vi "Encoder State.vi"(8 "error in (no error)":errorcluster) -> (0 "error out":errorcluster, 2 "Gamma":dbl, 3 "Combined Wheel Angle":dbl)   [LabVIEW 2014]
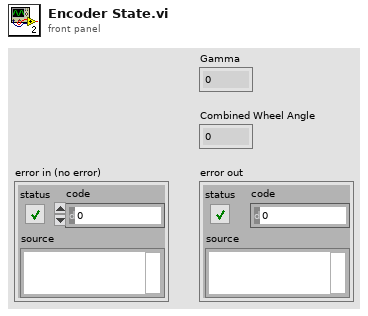
[diagram p1: front panel]
types:
  T1 = cluster{"Encoder 1":i32, "Encoder 2":i32, "Encoder 3":i32, "Encoder 4":i32}
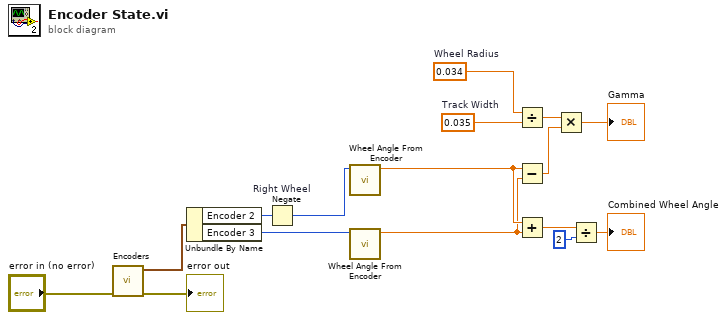
[diagram p0: block diagram]
diagram:
  w15 = 0.035  # Track Width
  w14 = 0.034  # Wheel Radius
  n1 = call "Encoders.vi"("error in (no error)"="error in (no error)") -> ("error out"=→"error out":errorcluster, "Encoder Data"=w3:T1)  [unwired: 9 in]
  n2 = Unbundle By Name(w3) -> ("Encoder 2"=w2:i32, "Encoder 3"=w1:i32)
  n3 = Negate "Right Wheel"(x=w2) -> (-x=w10:i32)
  n4 = call "Wheel Angle From Encoder.vi"("Numeric in"=w10) -> ("Numeric out"=w12:dbl)  [unwired: 10 in]
  n5 = call "Wheel Angle From Encoder.vi"("Numeric in"=w1) -> ("Numeric out"=w11:dbl)  [unwired: 10 in]
  n6 = Divide(x=w14, y=w15) -> (x/y=w16:dbl)
  n7 = Subtract(x=w12, y=w11) -> (x-y=w5:dbl)
  n8 = Add(x=w12, y=w11) -> (x+y=w7:dbl)
  n9 = Multiply(x=w16, y=w5) -> (x*y=→"Gamma":dbl)
  n10 = Divide(x=w7, y=2) -> (x/y=→"Combined Wheel Angle":dbl)
